vi "NMEA_ParseMessage-GPGGA.vi"(9 "Error In":errorcluster, 10 "$GPGGA-message_IN":string) -> (1 "Error Out":errorcluster, 2 "$GPGGA-message_OUT":T1={"TimeStamp"=timestamp(0 s since 1904-01-01), "Latitude"=0.0, "Latitude-Direction"=enum."", "Longitude"=1.0, "Longitude-Direction"=enum."", "GPS-Quality"=enum."GPS fix (SPS)", "Number of Satellites"=0, "Horizontal Dilution of Precision"=0.0, "Altitude above Mean-Sea-Level"=0.0, "Geoidal separation"=0.0, "Time since last DGPS update"=0.0, "DGPS reference station ID"=0} {"Time since last DGPS update" format="%.02f [s]"; "Geoidal separation" format="%.02f [m]"; "Altitude above Mean-Sea-Level" format="%.02f [m]"; "Horizontal Dilution of Precision" format="%.02f [HDOP]"; "Longitude" format="%0.4f [long]"; "Latitude" format="%.04f [lat]"; "TimeStamp" format="%<%.2X>T"})   [LabVIEW 2019, in "NMEA.lvlib"]
doc: "<B>GPGGA</B>\nGlobal Positioning System Fix Data"
uses:
  NMEA.lvlib
  NMEA_GPGGA-data.ctl
  NMEA_LatitudeDirection.ctl
  NMEA_LongitudeDirection.ctl
  NMEA_GPS-Quality.ctl
panel:
  out "x+y":timestamp
  in  "y":dbl
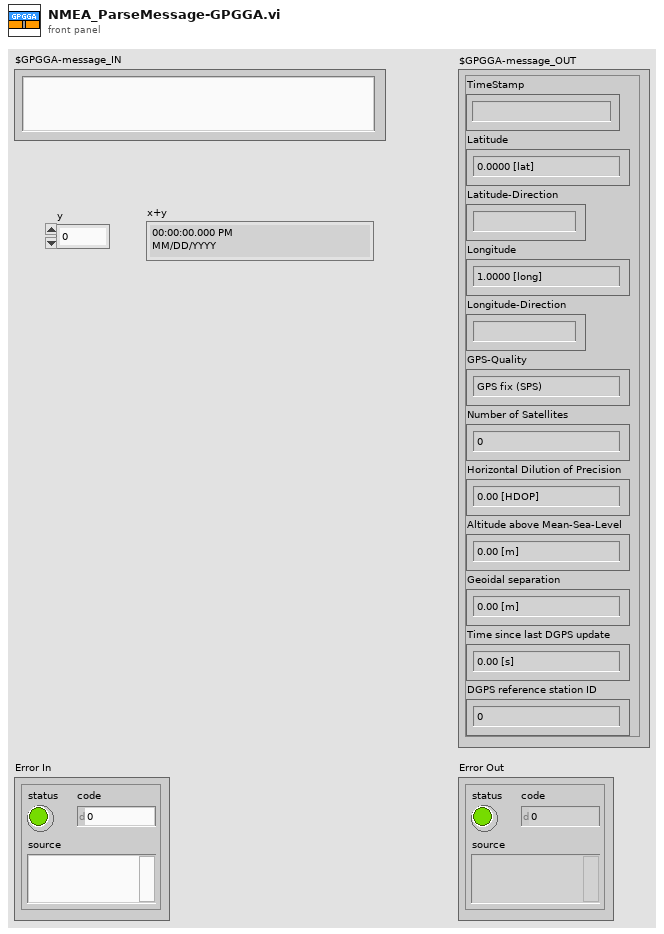
[diagram p1: front panel]
types:
  T1 = typedef "NMEA.lvlib/NMEA_GPGGA-data.ctl" = cluster{"TimeStamp":timestamp, "Latitude":dbl, "Latitude-Direction":T2, "Longitude":dbl, "Longitude-Direction":T3, "GPS-Quality":T4, "Number of Satellites":i32, "Horizontal Dilution of Precision":dbl, "Altitude above Mean-Sea-Level":dbl, "Geoidal separation":dbl, "Time since last DGPS update":dbl, "DGPS reference station ID":i32}
  T2 = typedef "NMEA.lvlib/NMEA_LatitudeDirection.ctl" = enum16{"", "North", "South"}
  T3 = typedef "NMEA.lvlib/NMEA_LongitudeDirection.ctl" = enum16{"", "East", "West"}
  T4 = typedef "NMEA.lvlib/NMEA_GPS-Quality.ctl" = enum16{"Invalid", "GPS fix (SPS)", "DGPS fix", "PPS fix", "Real Time Kinematic", "Float RTK", "estimated", "Manual input mode", "Simulation mode"}
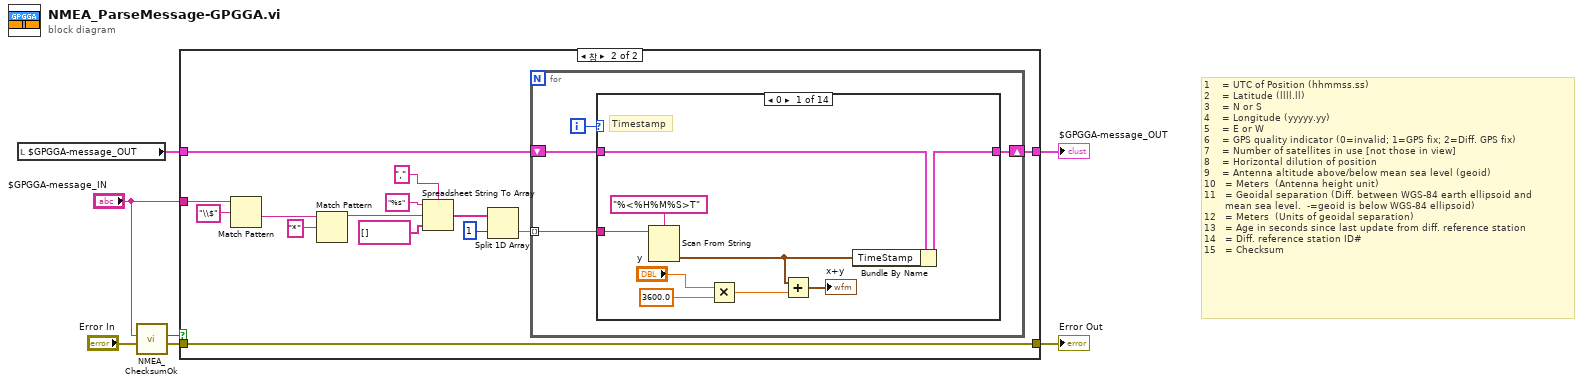
[diagram p0: block diagram]
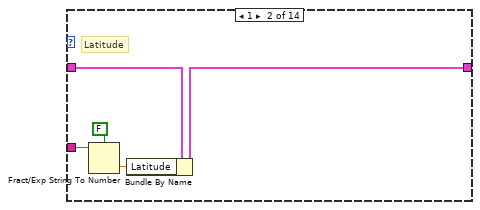
[diagram p3: hidden frame]
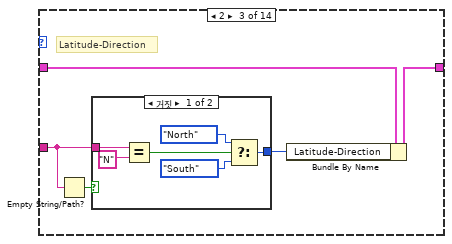
[diagram p4: hidden frame]
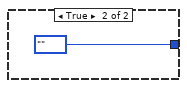
[diagram p5: hidden frame]
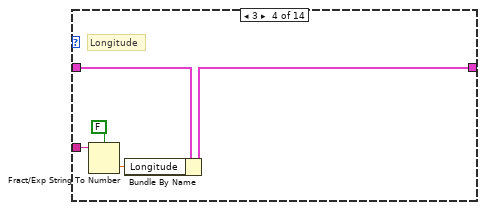
[diagram p6: hidden frame]
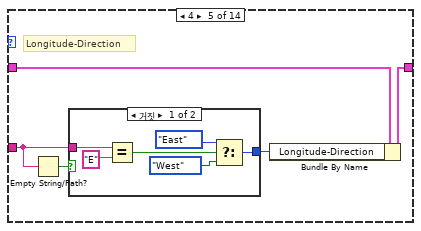
[diagram p7: hidden frame]
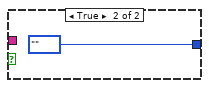
[diagram p8: hidden frame]
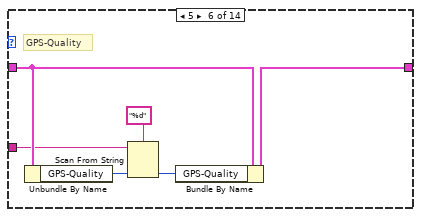
[diagram p9: hidden frame]
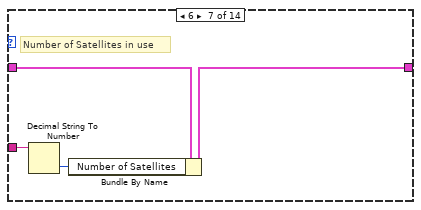
[diagram p10: hidden frame]
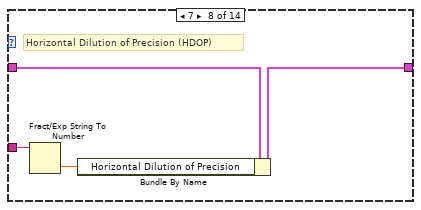
[diagram p11: hidden frame]
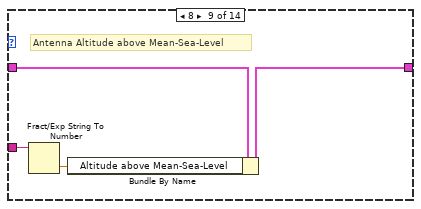
[diagram p12: hidden frame]
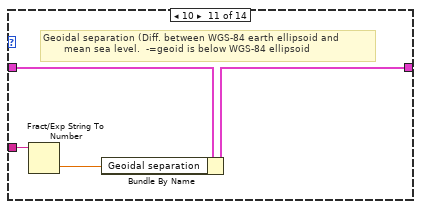
[diagram p14: hidden frame]
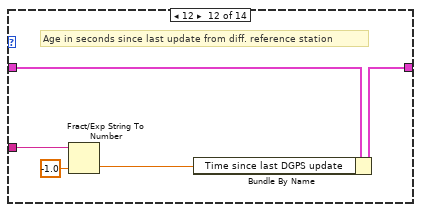
[diagram p15: hidden frame]
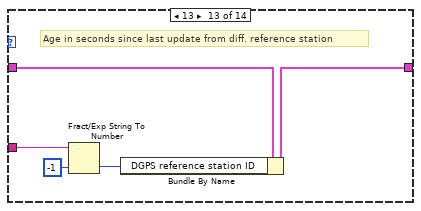
[diagram p16: hidden frame]
diagram:
  # "1    = UTC of Position (hhmmss.ss)\n2    = Latitude (llll.ll)\n3    = N or S\n4    = Longitude (yyyyy.yy)\n5    = E or W\n6    = GPS quality indicator (0=invalid; 1=GPS fix; 2=Diff. GPS fix)\n7    = Number of satellites in use [not those in view]\n8    = Horizontal dilution of position\n9    = Antenna altitude above/below mean sea level (geoid)\n10   = Meters  (Antenna height unit)\n11   = Geoidal separation (Diff. between WGS-84 earth ellipsoid and\n       mean sea level.  -=geoid is below WGS-84 ellipsoid)\n12   = Meters  (Units of geoidal separation)\n13   = Age in seconds since last update from diff. reference station\n14   = Diff. reference station ID#\n15   = Checksum"
  n1 = local read "$GPGGA-message_OUT"() -> (w7:T1)
  n2 = call "NMEA_ChecksumOk.vi"("Error In"="Error In", "Sentence"="$GPGGA-message_IN") -> ("Error Out"=w1:errorcluster, "CheckSumOk?"=w4:bool)  [unwired: 8 in]
  n3 = case shown="참" w4 {
    tunnel: w7 -> [w9 w18]
    tunnel: [w9 w17] -> w6
    tunnel: "$GPGGA-message_IN" -> [_ w15]
    tunnel: w1 -> [w8 w10]
    tunnel: [w8 w10] -> w3
    frame False {
    }
    frame True {
      n4 = Match Pattern(string=w15, regular expression="\\$") -> (after substring=w14:string)  [unwired: 1 in, 3 out]
      n5 = Match Pattern(string=w14, regular expression="*") -> (before substring=w22:string)  [unwired: 1 in, 3 out]
      n6 = Spreadsheet String To Array(delimiter (Tab)=",", format string="%s", spreadsheet string=w22, array type (2D Dbl)=string[] []) -> (array=w12:string[])
      n7 = Split 1D Array(array=w12, index=1) -> (second subarray=w13:string[])  [unwired: 1 out]
      n8 = for {
        tunnel: w13 -> [w24] mode=indexing
        shift-right: [w26] -> w17
        shift-left: w18 -> [w27]
        i -> [w25]
        n9 = case shown="0" w25 {
          tunnel: w27 -> [w36 w41 w46 w58 w63 w75 w80 w84 w88 w89 w93 w98 w103 w104]
          tunnel: [w35 w40 w45 w57 w62 w76 w79 w83 w87 w89 w92 w97 w102 w104] -> w26
          tunnel: w24 -> [w33 w39 w43 w56 w60 w72 w78 w82 w86 _ w91 w96 w101 _]
          frame 0 {
            # "Timestamp"
            n10 = Scan From String(format string="%<%H%M%S>T", input string=w33) -> (output 1=w32:timestamp)  [unwired: 3 in, 3 out]
            n11 = Multiply(x="y", y=3600.0) -> (x*y=w29:dbl)
            n12 = Add(x=w32, y=w29) -> (x+y=→"x+y":timestamp)
            n13 = Bundle By Name(cluster=w36, "TimeStamp"=w32) -> (w35:T1)
          }
          frame 1 {
            # "Latitude"
            n14 = Fract/Exp String To Number(use system decimal point (T)=FALSE, string=w39) -> (number=w38:dbl)  [unwired: 2 in, 1 out]
            n15 = Bundle By Name(cluster=w41, "Latitude"=w38) -> (w40:T1)
          }
          frame 2 {
            # "Latitude-Direction"
            n16 = Empty String/Path?(string/path=w43) -> (empty?=w42:bool)
            n17 = case shown="거짓" w42 {
              tunnel: [w49 NMEA_LatitudeDirection."" ("f")] -> w44
              tunnel: w43 -> [w47 _]
              frame False {
                n18 = Equal?(x=w47, y="N") -> (x = y?=w51:bool)
                n19 = Select(t=NMEA_LatitudeDirection."North" ("Latitude-Direction"), s=w51, f=NMEA_LatitudeDirection."South") -> (s? t:f=w49:T2)
              }
              frame True {
              }
            }
            n20 = Bundle By Name(cluster=w46, "Latitude-Direction"=w44) -> (w45:T1)
          }
          frame 3 {
            # "Longitude"
            n21 = Fract/Exp String To Number(use system decimal point (T)=FALSE, string=w56) -> (number=w55:dbl)  [unwired: 2 in, 1 out]
            n22 = Bundle By Name(cluster=w58, "Longitude"=w55) -> (w57:T1)
          }
          frame 4 {
            # "Longitude-Direction"
            n23 = Empty String/Path?(string/path=w60) -> (empty?=w59:bool)
            n24 = case shown="거짓" w59 {
              tunnel: w60 -> [w69 _]
              tunnel: [w65 NMEA_LongitudeDirection."" ("f")] -> w61
              frame False {
                n25 = Equal?(x=w69, y="E") -> (x = y?=w67:bool)
                n26 = Select(t=NMEA_LongitudeDirection."East" ("Longitude-Direction"), s=w67, f=NMEA_LongitudeDirection."West") -> (s? t:f=w65:T3)
              }
              frame True {
              }
            }
            n27 = Bundle By Name(cluster=w63, "Longitude-Direction"=w61) -> (w62:T1)
          }
          frame 5 {
            # "GPS-Quality"
            n28 = Unbundle By Name(w75) -> ("GPS-Quality"=w74:T4)
            n29 = Scan From String(format string="%d", input string=w72, default 1=w74) -> (output 1=w73:T4)  [unwired: 2 in, 3 out]
            n30 = Bundle By Name(cluster=w75, "GPS-Quality"=w73) -> (w76:T1)
          }
          frame 6 {
            # "Number of Satellites in use"
            n31 = Decimal String To Number(string=w78) -> (number=w77:i32)  [unwired: 2 in, 1 out]
            n32 = Bundle By Name(cluster=w80, "Number of Satellites"=w77) -> (w79:T1)
          }
          frame 7 {
            # "Horizontal Dilution of Precision (HDOP)"
            n33 = Fract/Exp String To Number(string=w82) -> (number=w81:dbl)  [unwired: 3 in, 1 out]
            n34 = Bundle By Name(cluster=w84, "Horizontal Dilution of Precision"=w81) -> (w83:T1)
          }
          frame 8 {
            # "Antenna Altitude above Mean-Sea-Level"
            n35 = Fract/Exp String To Number(string=w86) -> (number=w85:dbl)  [unwired: 3 in, 1 out]
            n36 = Bundle By Name(cluster=w88, "Altitude above Mean-Sea-Level"=w85) -> (w87:T1)
          }
          frame 9, 11 {
            # "[9] - Meters (antenna height unit)\n[11] - Meters (units of geoidal separation)"
          }
          frame 10 {
            # "Geoidal separation (Diff. between WGS-84 earth ellipsoid and\n       mean sea level.  -=geoid is below WGS-84 ellipsoid"
            n37 = Fract/Exp String To Number(string=w91) -> (number=w90:dbl)  [unwired: 3 in, 1 out]
            n38 = Bundle By Name(cluster=w93, "Geoidal separation"=w90) -> (w92:T1)
          }
          frame 12 {
            # "Age in seconds since last update from diff. reference station"
            n39 = Fract/Exp String To Number(string=w96, default (0 dbl)=-1.0 ("default (0 DBL)")) -> (number=w95:dbl)  [unwired: 2 in, 1 out]
            n40 = Bundle By Name(cluster=w98, "Time since last DGPS update"=w95) -> (w97:T1)
          }
          frame 13 {
            # "Age in seconds since last update from diff. reference station"
            n41 = Fract/Exp String To Number(string=w101, default (0 dbl)=-1 ("DGPS reference station ID")) -> (number=w100:i32)  [unwired: 2 in, 1 out]
            n42 = Bundle By Name(cluster=w103, "DGPS reference station ID"=w100) -> (w102:T1)
          }
          frame Default {
          }
        }
      }
    }
  }
  "$GPGGA-message_OUT" <- w6
  "Error Out" <- w3
